vi "FVIR Button Disable.vi"(7 "UI Refs":T5, 8 "error in (no error)":errorcluster, 10 "PLC Data In":T1, 11 "Queue in":refnum<queue>) -> (0 "error out":errorcluster, 2 "PLC Data Out":T1, 3 "Queue out":refnum<queue>)   [LabVIEW 2020]
uses:
  Message Queue/Message Cluster.ctl
  controls/UI Data.ctl
  Modbus/Modbus PLC Data All.ctl
  Modbus/Modbus FVIR Control.ctl
  Modbus/Modbus LDO Control.ctl
  WritingDataFile/Data to Save.ctl
  Message Queue/Enqueue Message (Single).vi
  Message Queue/Message Queue.lvlib
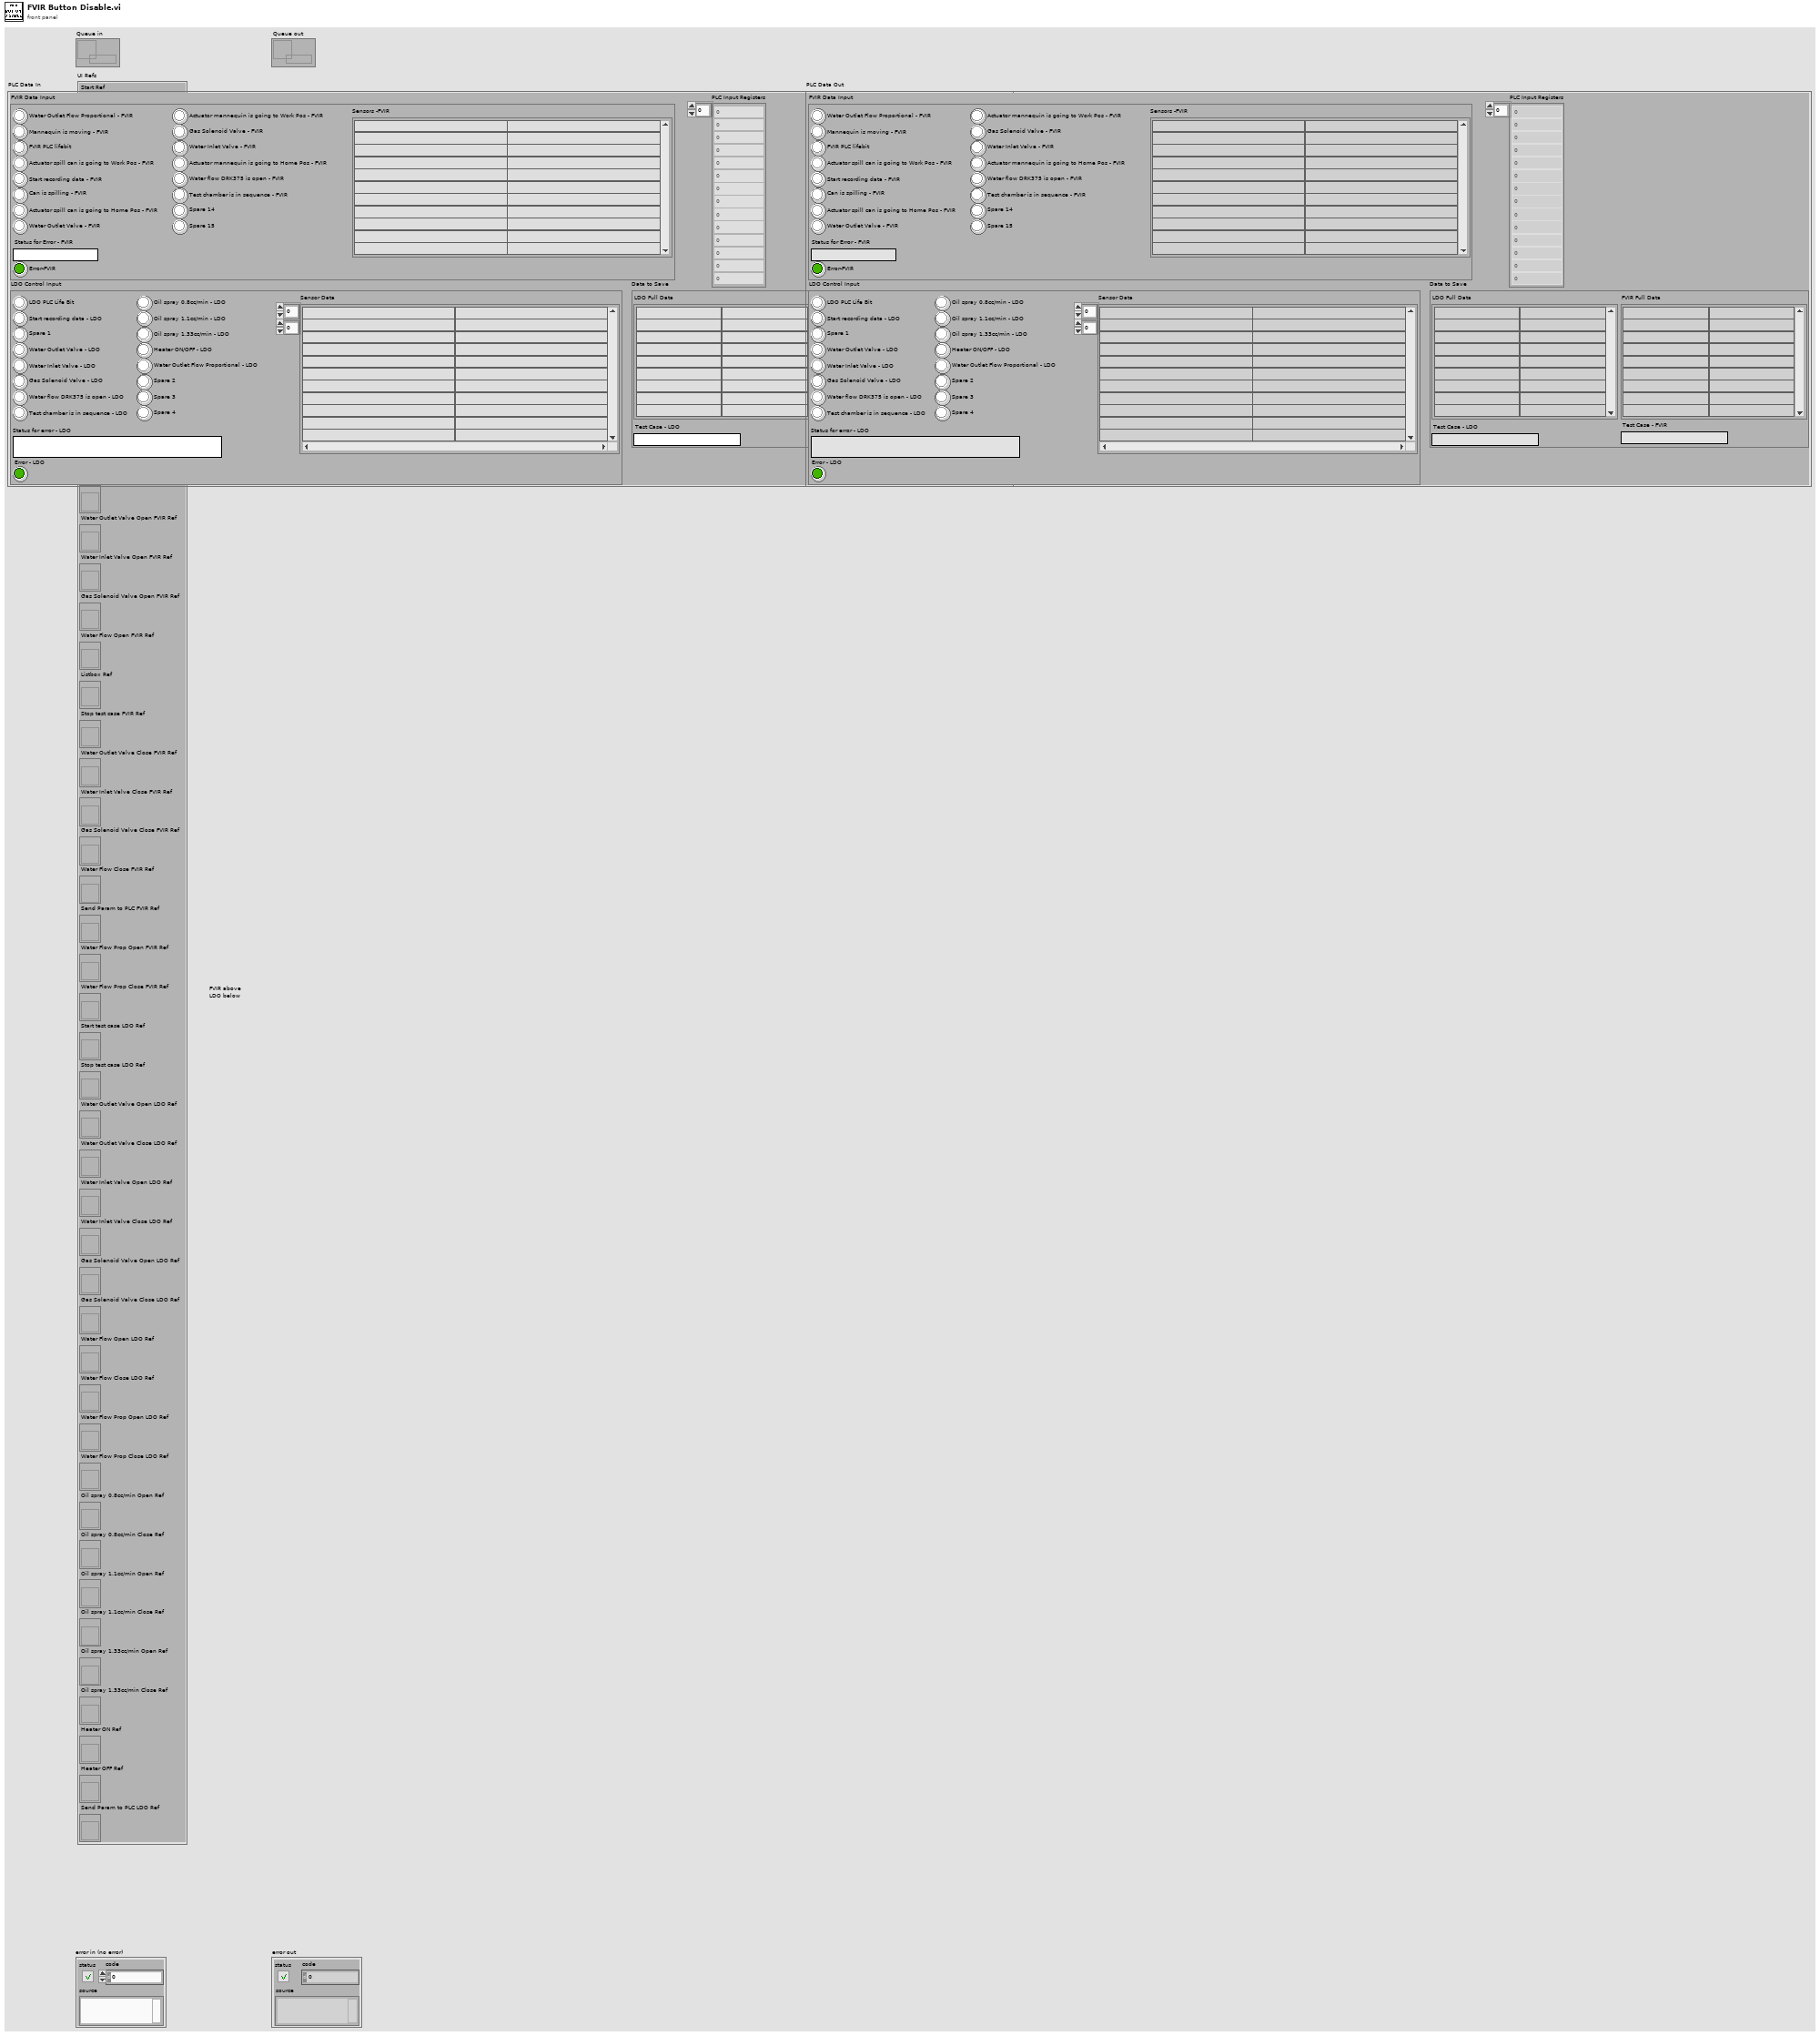
[diagram p1: front panel]
types:
  T1 = typedef "Modbus PLC Data All.ctl" = cluster{"FVIR Data Input":T2, "LDO Control Input":T3, "PLC Input Registers":u16[], "Data to Save":T4}
  T2 = typedef "Modbus FVIR Control.ctl" = cluster{"Spare 15":bool, "Spare 14":bool, "Actuator mannequin is going to Work Pos - FVIR":bool, "Actuator mannequin is going to Home Pos - FVIR":bool, "Test chamber is in sequence - FVIR ":bool, "Water flow DRK375 is open - FVIR":bool, "Gas Solenoid Valve - FVIR":bool, "Water Inlet Valve - FVIR":bool, "Water Outlet Flow Proportional - FVIR":bool, "Start recording data - FVIR":bool, "Actuator spill can is going to Work Pos - FVIR":bool, "Actuator spill can is going to Home Pos - FVIR":bool, "Water Outlet Valve - FVIR":bool, "Can is spilling - FVIR":bool, "Mannequin is moving - FVIR":bool, "FVIR PLC lifebit":bool, "Status for Error - FVIR":string, "Error-FVIR":bool, "Sensors -FVIR":string[][]}
  T3 = typedef "Modbus LDO Control.ctl" = cluster{"LDO PLC Life Bit":bool, "Start recording data - LDO":bool, "Spare 1":bool, "Water Outlet Valve - LDO":bool, "Water Inlet Valve - LDO":bool, "Gas Solenoid Valve - LDO":bool, "Water flow DRK375 is open - LDO":bool, "Test chamber is in sequence - LDO":bool, "Oil spray 0.8cc/min - LDO":bool, "Oil spray 1.1cc/min - LDO":bool, "Oil spray 1.33cc/min - LDO":bool, "Heater ON/OFF - LDO":bool, "Water Outlet Flow Proportional - LDO":bool, "Spare 2":bool, "Spare 3":bool, "Spare 4":bool, "Status for error - LDO":string, "Error - LDO":bool, "Sensor Data":string[][]}
  T4 = typedef "Data to Save.ctl" = cluster{"LDO Full Data":string[][], "FVIR Full Data":string[][], "Test Case - FVIR":string, "Test Case - LDO":string}
  T5 = typedef "UI Data.ctl" = cluster{"Start Ref":refnum<vi>, "Stop Ref":refnum<vi>, "Exit Ref":refnum<vi>, "Status Ref":refnum<vi>, "Connect Ref":refnum<vi>, "Disconnect Ref":refnum<vi>, "Spill can Home pos Ref":refnum<vi>, "Spill can Work pos Ref":refnum<vi>, "Move Mannequin Home pos Ref":refnum<vi>, "Move Mannequin Work pos Ref":refnum<vi>, "Start test case FVIR Ref":refnum<vi>, "Water Outlet Valve Open FVIR Ref":refnum<vi>, "Water Inlet Valve Open FVIR Ref":refnum<vi>, "Gas Solenoid Valve Open FVIR Ref":refnum<vi>, "Water Flow Open FVIR Ref":refnum<vi>, "Listbox Ref":refnum<vi>, "Stop test case FVIR Ref":refnum<vi>, "Water Outlet Valve Close FVIR Ref":refnum<vi>, "Water Inlet Valve Close FVIR Ref":refnum<vi>, "Gas Solenoid Valve Close FVIR Ref":refnum<vi>, "Water Flow Close FVIR Ref":refnum<vi>, "Send Param to PLC FVIR Ref":refnum<vi>, "Water Flow Prop Open FVIR Ref":refnum<vi>, "Water Flow Prop Close FVIR Ref":refnum<vi>, "Start test case LDO Ref":refnum<vi>, "Stop test case LDO Ref":refnum<vi>, "Water Outlet Valve Open LDO Ref":refnum<vi>, "Water Outlet Valve Close LDO Ref":refnum<vi>, "Water Inlet Valve Open LDO Ref":refnum<vi>, "Water Inlet Valve Close LDO Ref":refnum<vi>, "Gas Solenoid Valve Open LDO Ref":refnum<vi>, "Gas Solenoid Valve Close LDO Ref":refnum<vi>, "Water Flow Open LDO Ref":refnum<vi>, "Water Flow Close LDO Ref":refnum<vi>, "Water Flow Prop Open LDO Ref":refnum<vi>, "Water Flow Prop Close LDO Ref":refnum<vi>, "Oil spray 0.8cc/min Open Ref":refnum<vi>, "Oil spray 0.8cc/min Close Ref":refnum<vi>, "Oil spray 1.1cc/min Open Ref":refnum<vi>, "Oil spray 1.1cc/min Close Ref":refnum<vi>, "Oil spray 1.33cc/min Open Ref":refnum<vi>, "Oil spray 1.33cc/min Close Ref":refnum<vi>, "Heater ON Ref":refnum<vi>, "Heater OFF Ref":refnum<vi>, "Send Param to PLC LDO Ref":refnum<vi>}
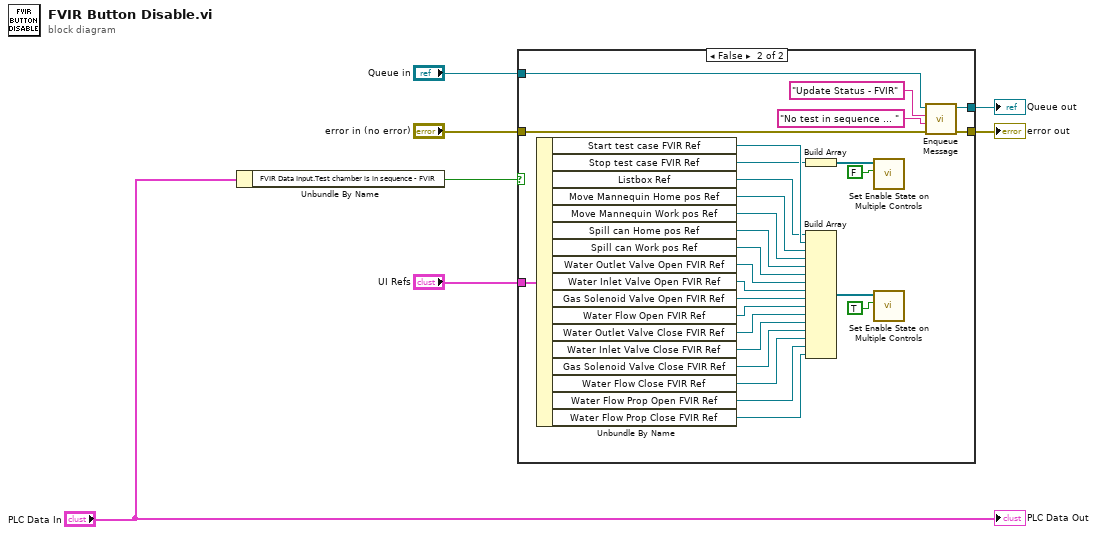
[diagram p0: block diagram]
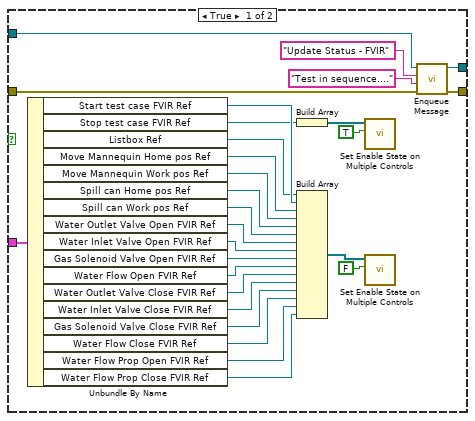
[diagram p2: hidden frame]
diagram:
  n1 = Unbundle By Name("PLC Data In") -> ("FVIR Data Input.Test chamber is in sequence - FVIR"=w1:bool)
  n2 = case shown="False" w1 {
    tunnel: "UI Refs" -> [w34 w62]
    tunnel: "Queue in" -> [w21 w49]
    tunnel: "error in (no error)" -> [w19 w47]
    tunnel: [w18 w46] -> w6
    tunnel: [w8 w36] -> w7
    frame True {
      n3 = Unbundle By Name(w34) -> ("Start test case FVIR Ref"=w17:refnum<vi>, "Stop test case FVIR Ref"=w16:refnum<vi>, "Listbox Ref"=w15:refnum<vi>, "Move Mannequin Home pos Ref"=w31:refnum<vi>, "Move Mannequin Work pos Ref"=w30:refnum<vi>, "Spill can Home pos Ref"=w29:refnum<vi>, "Spill can Work pos Ref"=w28:refnum<vi>, "Water Outlet Valve Open FVIR Ref"=w27:refnum<vi>, "Water Inlet Valve Open FVIR Ref"=w26:refnum<vi>, "Gas Solenoid Valve Open FVIR Ref"=w25:refnum<vi>, "Water Flow Open FVIR Ref"=w24:refnum<vi>, "Water Outlet Valve Close FVIR Ref"=w14:refnum<vi>, "Water Inlet Valve Close FVIR Ref"=w13:refnum<vi>, "Gas Solenoid Valve Close FVIR Ref"=w12:refnum<vi>, "Water Flow Close FVIR Ref"=w11:refnum<vi>, "Water Flow Prop Open FVIR Ref"=w10:refnum<vi>, "Water Flow Prop Close FVIR Ref"=w9:refnum<vi>)
      n4 = Build Array(w16) -> (w32:refnum<vi>[])
      n5 = Build Array(w15, w17, w31, w30, w29, w28, w27, w26, w25, w24, w14, w13, w12, w11, w10, w9) -> (w23:refnum<vi>[])
      n6 = call "Set Enable State on Multiple Controls.vi"("Enable?"=TRUE, "Controls"=w32) -> ()  [unwired: 10 in]
      n7 = call "Set Enable State on Multiple Controls.vi"("Enable?"=FALSE, "Controls"=w23) -> ()  [unwired: 10 in]
      n8 = call-poly "Enqueue Message.vi"("error in (no error)"=w19, "Message Data"="Test in sequence...." ("Acquiring and Logging..."), "Message"="Update Status - FVIR", "Message Queue"=w21) -> ("error out"=w18:errorcluster, "dup Message Queue"=w8:refnum<queue>)  [unwired: 6 in]
    }
    frame False {
      n9 = Unbundle By Name(w62) -> ("Start test case FVIR Ref"=w45:refnum<vi>, "Stop test case FVIR Ref"=w44:refnum<vi>, "Listbox Ref"=w43:refnum<vi>, "Move Mannequin Home pos Ref"=w59:refnum<vi>, "Move Mannequin Work pos Ref"=w58:refnum<vi>, "Spill can Home pos Ref"=w57:refnum<vi>, "Spill can Work pos Ref"=w56:refnum<vi>, "Water Outlet Valve Open FVIR Ref"=w55:refnum<vi>, "Water Inlet Valve Open FVIR Ref"=w54:refnum<vi>, "Gas Solenoid Valve Open FVIR Ref"=w53:refnum<vi>, "Water Flow Open FVIR Ref"=w52:refnum<vi>, "Water Outlet Valve Close FVIR Ref"=w42:refnum<vi>, "Water Inlet Valve Close FVIR Ref"=w41:refnum<vi>, "Gas Solenoid Valve Close FVIR Ref"=w40:refnum<vi>, "Water Flow Close FVIR Ref"=w39:refnum<vi>, "Water Flow Prop Open FVIR Ref"=w38:refnum<vi>, "Water Flow Prop Close FVIR Ref"=w37:refnum<vi>)
      n10 = Build Array(w44) -> (w60:refnum<vi>[])
      n11 = Build Array(w43, w45, w59, w58, w57, w56, w55, w54, w53, w52, w42, w41, w40, w39, w38, w37) -> (w51:refnum<vi>[])
      n12 = call "Set Enable State on Multiple Controls.vi"("Enable?"=FALSE, "Controls"=w60) -> ()  [unwired: 10 in]
      n13 = call "Set Enable State on Multiple Controls.vi"("Enable?"=TRUE, "Controls"=w51) -> ()  [unwired: 10 in]
      n14 = call-poly "Enqueue Message.vi"("error in (no error)"=w47, "Message Data"="No test in sequence ... " ("Acquiring and Logging..."), "Message"="Update Status - FVIR", "Message Queue"=w49) -> ("error out"=w46:errorcluster, "dup Message Queue"=w36:refnum<queue>)  [unwired: 6 in]
    }
  }
  "Queue out" <- w7
  "error out" <- w6
  "PLC Data Out" <- "PLC Data In"
